vi "Set SDI Address.vi"(8 "error in (no error)":errorcluster, 10 "SDI Address":string, 11 "H3611i Actor in":refnum<class "H3611i Actor.lvclass">) -> (0 "error out":errorcluster, 3 "H3611i Actor out":refnum<class "H3611i Actor.lvclass">)   [LabVIEW 2018, in "H3611i.lvlib" / "H3611i Actor.lvclass"]
uses:
  H3611i Actor.lvclass
  C:/Users/dev/Documents/CODE/LabVIEW/microwaveverify/trunk/MWWL Verification/Sensor Actor/Sensor/Sensor.lvclass
  H3611i Actor.lvclass/H3611i Actor.ctl
  Sensor Actor/Sensor/Sensor.lvclass
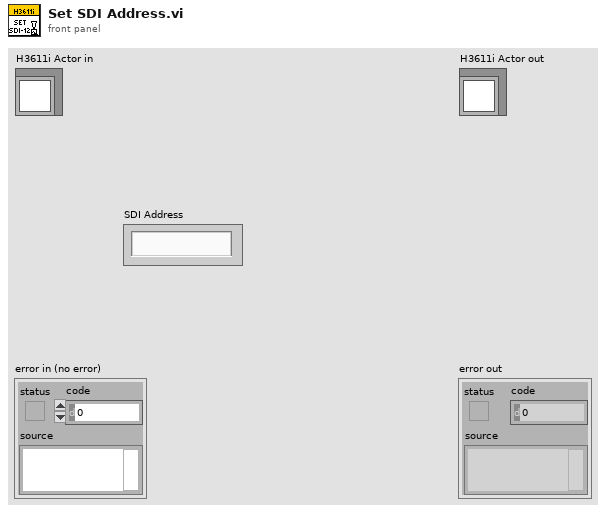
[diagram p1: front panel]
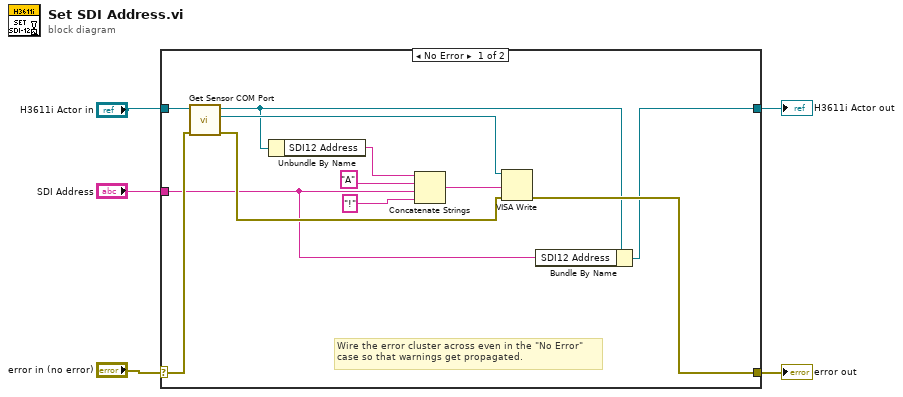
[diagram p0: block diagram]
diagram:
  n1 = case shown="No Error" "error in (no error)" {
    selector: "error in (no error)" -> [w16 w19]
    tunnel: [w9 w19] -> w4
    tunnel: [w6 w18] -> w2
    tunnel: "H3611i Actor in" -> [w17 w18]
    tunnel: "SDI Address" -> [w8 _]
    frame No Error {
      # "Wire the error cluster across even in the \"No Error\"\ncase so that warnings get propagated."
      n2 = call "Get Sensor COM Port.vi"("error in (no error)"=w16, "Sensor in"=w17) -> ("error out"=w10:errorcluster, "COM Port"=w11:refnum<visa-resource-name>, "Sensor out"=w7:refnum<class "H3611i Actor.lvclass">)  [unwired: 7 in]
      n3 = Unbundle By Name(w7) -> ("SDI12 Address"=w14:string)
      n4 = Concatenate Strings(w14, "A", w8, "!" ("string")) -> (w13:string)
      n5 = VISA Write(VISA resource name=w11, write buffer=w13, error in (no error)=w10) -> (error out=w9:errorcluster)  [unwired: 2 out]
      n6 = Bundle By Name(cluster=w7, "SDI12 Address"=w8) -> (w6:refnum<class "H3611i Actor.lvclass">)
    }
    frame Error {
    }
  }
  "error out" <- w4
  "H3611i Actor out" <- w2
